vi "Philosophers FP.PanelBounds.vi"(8 "error in":errorcluster, 10 "# Philosophers":i32, 11 "Philospoher":i32) -> (0 "error out":errorcluster, 3 "Location chair":T1)   [LabVIEW 2021, in "Table.lvclass"]
doc: "Positiion Philosopher on screen"
uses:
  Table.lvclass
  <vilib>/Utility/miscctls.llb/LVRectTypeDef.ctl
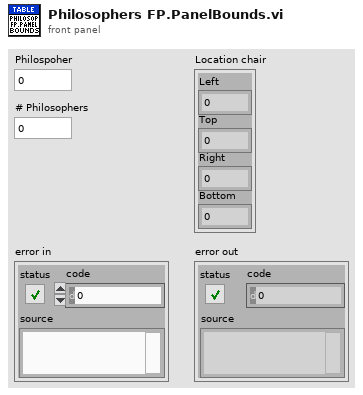
[diagram p1: front panel]
types:
  T1 = typedef "LVRectTypeDef.ctl" = cluster{"Left":i16, "Top":i16, "Right":i16, "Bottom":i16}
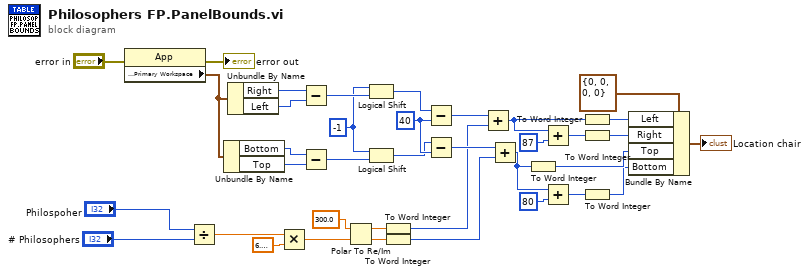
[diagram p0: block diagram]
diagram:
  w23 = i16 -1 ("y")
  w35 = i16 40 ("y")
  n1 = property on="Property Node" class="App"(error in="error in") -> (error out=→"error out":errorcluster, "Display:Primary Workspace"=w29:T1)  [unwired: 1 in, 1 out]
  n2 = Divide(x="Philospoher", y="# Philosophers") -> (x/y=w22:dbl)
  n3 = Unbundle By Name(w29) -> ("Bottom"=w31:i16, "Top"=w32:i16)
  n4 = Unbundle By Name(w29) -> ("Right"=w26:i16, "Left"=w27:i16)
  n5 = Multiply(x=w22, y=6.283185307179586 ("Pi Multiplied By 2")) -> (x*y=w20:dbl)
  n6 = Subtract(x=w26, y=w27) -> (x-y=w28:i16)
  n7 = Subtract(x=w31, y=w32) -> (x-y=w30:i16)
  n8 = Polar To Re/Im(2:w20, 3:300.0 ("r")) -> (0:w17:dbl, 1:w18:dbl)
  n9 = Logical Shift(y=w23, x=w28) -> (x << y=w25:i16)
  n10 = Logical Shift(y=w23, x=w30) -> (x << y=w24:i16)
  n11 = To Word Integer(number=w18) -> (16bit integer=w3:i16)
  n12 = To Word Integer(number=w17) -> (16bit integer=w2:i16)
  n13 = Subtract(x=w25, y=w35) -> (x-y=w33:i16)
  n14 = Subtract(x=w24, y=w35) -> (x-y=w34:i16)
  n15 = Add(x=w33, y=w3) -> (x+y=w15:i16)
  n16 = Add(x=w34, y=w2) -> (x+y=w11:i16)
  n17 = To Word Integer(number=w11) -> (16bit integer=w7:i16)
  n18 = Add(x=w15, y=i16 87) -> (x+y=w10:i16)
  n19 = Add(x=w11, y=i16 80) -> (x+y=w13:i16)
  n20 = To Word Integer(number=w15) -> (16bit integer=w9:i16)
  n21 = To Word Integer(number=w10) -> (16bit integer=w8:i16)
  n22 = To Word Integer(number=w13) -> (16bit integer=w6:i16)
  n23 = Bundle By Name(cluster=T1 {"Left"=0, "Top"=0, "Right"=0, "Bottom"=0} ("Front Panel Window:Window Bounds"), "Left"=w9, "Right"=w8, "Top"=w7, "Bottom"=w6) -> (→"Location chair":T1)
